vi "Acquisition Done.vi"(8 "error in (no error)":errorcluster, 11 "Cam_SLM_Controller in":refnum<class "Cam_SLM_Controller.lvclass">) -> (0 "error out":errorcluster, 3 "Cam_SLM_Controller out":refnum<class "Cam_SLM_Controller.lvclass">)   [LabVIEW 2023, in "Cam_SLM_controller.lvlib" / "Cam_SLM_Controller.lvclass"]
uses:
  Cam_SLM_Controller.lvclass
  Cam_SLM_Controller.lvclass/Cam_SLM_Controller.ctl
  UIs/SLM_Controller/SLM_Controller/SLM_Controller Messages/Upload Next Msg/Upload Next Msg.lvclass/Upload Next Msg.ctl
  <vilib>/ActorFramework/Message Enqueuer/Message Enqueuer.lvclass/Message Enqueuer.ctl
  <vilib>/ActorFramework/Message Enqueuer/Enqueue.vi
  UIs/SLM_Controller/SLM_Controller/SLM_Controller Messages/Upload Next Msg/Upload Next Msg.lvclass
  C:/Program Files/National Instruments/LabVIEW 2023/vi.lib/ActorFramework/Message/Message.lvclass
  UIs/SLM_Controller/SLM_Controller/SLM_Controller Messages/Scan Done Msg/Scan Done Msg.lvclass
  <vilib>/ActorFramework/Message Priority Queue/Priority Enqueue.vi
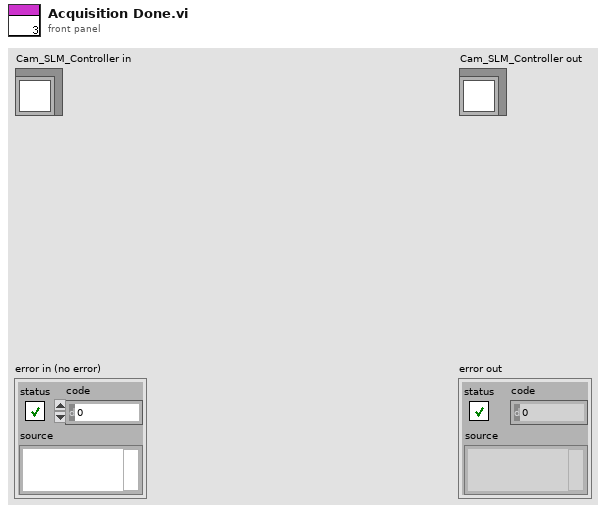
[diagram p1: front panel]
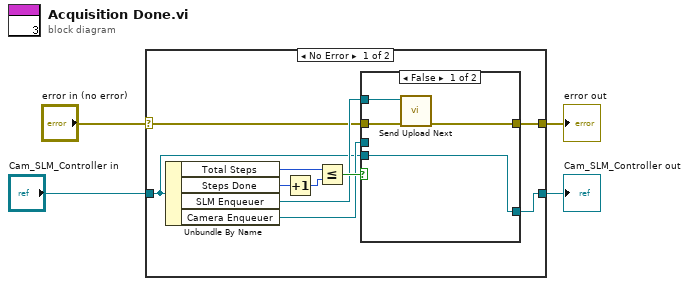
[diagram p0: block diagram]
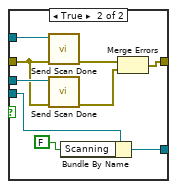
[diagram p2: hidden frame]
diagram:
  n1 = case shown="No Error" "error in (no error)" {
    selector: "error in (no error)" -> [w8 w29]
    tunnel: [w7 w29] -> w3
    tunnel: [w5 w28] -> w1
    tunnel: "Cam_SLM_Controller in" -> [w6 w28]
    frame No Error {
      n2 = Unbundle By Name(w6) -> ("Total Steps"=w12:u16, "Steps Done"=w14:u16, "SLM Enqueuer"=w10:refnum<class "Message Enqueuer.lvclass">, "Camera Enqueuer"=w9:refnum<class "Message Enqueuer.lvclass">)
      n3 = Increment(x=w14) -> (x+1=w13:u16)
      n4 = Less Or Equal?(x=w12, y=w13) -> (x <= y?=w11:bool)
      n5 = case shown="False" w11 {
        tunnel: w10 -> [w16 w27]
        tunnel: w9 -> [_ w26]
        tunnel: w8 -> [w17 w25]
        tunnel: [w18 w22] -> w7
        tunnel: w6 -> [w15 w21]
        tunnel: [w15 w20] -> w5
        frame False {
          n6 = call "Send Upload Next.vi"("error in (no error)"=w17, "Message Enqueuer"=w16) -> ("error out"=w18:errorcluster)  [unwired: 8 in, 1 out]
        }
        frame True {
          n7 = call "Send Scan Done.vi"("error in (no error)"=w25, "Message Enqueuer"=w27) -> ("error out"=w24:errorcluster)  [unwired: 8 in, 1 out]
          n8 = call "Send Scan Done.vi"("error in (no error)"=w25, "Message Enqueuer"=w26) -> ("error out"=w23:errorcluster)  [unwired: 8 in, 1 out]
          n9 = Bundle By Name(cluster=w21, "Scanning"=FALSE) -> (w20:refnum<class "Cam_SLM_Controller.lvclass">)
          n10 = Merge Errors(w24, w23) -> (w22:errorcluster)
        }
      }
    }
    frame Error {
    }
  }
  "error out" <- w3
  "Cam_SLM_Controller out" <- w1
